vi "get_specification.vi"(8 "error in (no error)":errorcluster, 11 "GenericPlugin in":refnum<class "GenericComponent.lvclass">) -> (0 "error out":errorcluster, 2 "component specification":T1, 3 "GenericPlugin out":refnum<class "GenericComponent.lvclass">, 4 "settings specified?":bool)   [LabVIEW 2010, in "GenericComponent.lvclass"]
uses:
  GenericComponent.lvclass
  clusters/plugin_specification.ctl
  GenericComponent.lvclass/GenericComponent.ctl
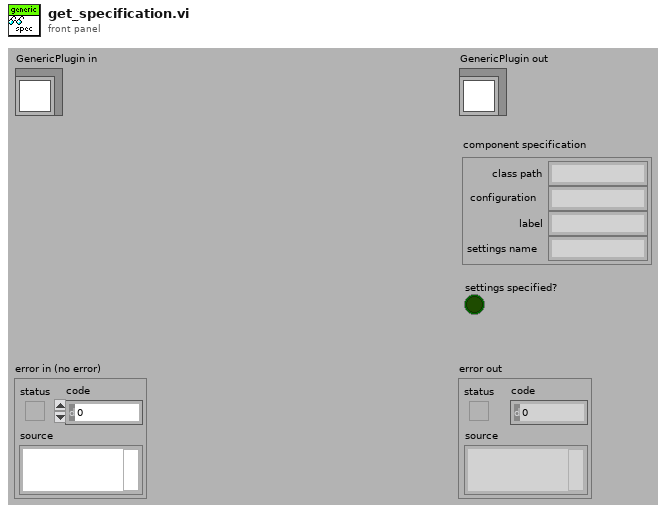
[diagram p1: front panel]
types:
  T1 = typedef "plugin_specification.ctl" = cluster{"class path":string, "configuration":string, "label":string, "settings name":string}
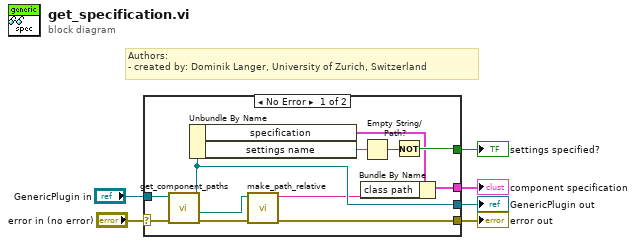
[diagram p0: block diagram]
diagram:
  # "Authors: \n- created by: Dominik Langer, University of Zurich, Switzerland"
  n1 = case shown="No Error" "error in (no error)" {
    selector: "error in (no error)" -> [w15 w19]
    tunnel: [w9 w19] -> w5
    tunnel: [w11 w20] -> w3
    tunnel: "GenericPlugin in" -> [w14 w20]
    tunnel: [w12 _] -> w2
    tunnel: [w16 _] -> w1
    frame No Error {
      n2 = call-dynamic "get_component_paths.vi"("error in (no error)"=w15, "GenericComponent in"=w14) -> ("error out"=w10:errorcluster, "component class path"=w8:path, "GenericComponent out"=w11:refnum<class "GenericComponent.lvclass">)  [unwired: 4 in, 3 out]
      n3 = Unbundle By Name(w11) -> ("specification"=w13:T1, "settings name"=w18:string)
      n4 = call "make_path_relative.vi"("error in (no error)"=w10, "absolute path"=w8) -> ("error out"=w9:errorcluster, "relative path"=w7:string)  [unwired: 8 in]
      n5 = Bundle By Name(cluster=w13, "class path"=w7) -> (w12:T1)
      n6 = Empty String/Path?(string/path=w18) -> (empty?=w17:bool)
      n7 = Not(x=w17) -> (.not. x?=w16:bool)
    }
    frame Error {
    }
  }
  "error out" <- w5
  "GenericPlugin out" <- w3
  "component specification" <- w2
  "settings specified?" <- w1
